vi "qTLT.vi"(0 "System no.":i32=1 min=1 max=4 step=1, 5 "error in":errorcluster) -> (14 "Number of tables":i32, 19 "error out":errorcluster)   [LabVIEW 2026]
doc: "Returns the number of DDL tables available in the controller."
panel:
  # "Returns the number of DDL tables available in the controller."
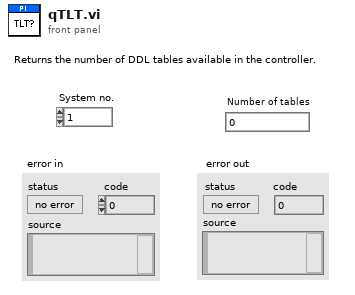
[diagram p1: front panel]
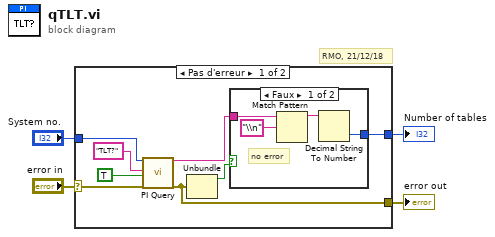
[diagram p0: block diagram]
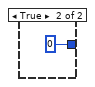
[diagram p2: hidden frame]
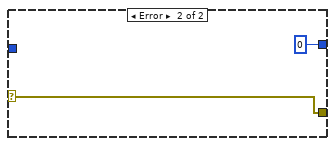
[diagram p3: hidden frame]
diagram:
  # "RMO, 21/12/18"
  n1 = case shown="Pas d'erreur" "error in" {
    selector: "error in" -> [w7 w18]
    tunnel: [w11 0] -> w4
    tunnel: [w6 w18] -> w3
    tunnel: "System no." -> [w9 _]
    frame No Error {
      n2 = call "PI Query.vi"("System no."=w9, "String to send"="TLT?", "Attach termination char.?"=TRUE ("Attach Linefeed?"), "error in"=w7) -> ("String read"=w5:string, "error out"=w6:errorcluster)  [unwired: 3 in, 11 out]
      n3 = Unbundle(w6) -> ("status"=w12:bool)  [unwired: 2 out]
      n4 = case shown="Faux" w12 {
        tunnel: w5 -> [w15 _]
        tunnel: [w16 0] -> w11
        frame False {
          # "no error"
          n5 = Match Pattern(string=w15, regular expression="\\n") -> (before substring=w13:string)  [unwired: 4 out]
          n6 = Decimal String To Number(string=w13) -> (number=w16:i32)  [unwired: 3 out]
        }
        frame True {
        }
      }
    }
    frame Error {
    }
  }
  "error out" <- w3
  "Number of tables" <- w4
